vi "settle timer.vi"(2 "in settle band":bool, 7 "Control Parameters":T1={"Setpoint"=50.0, "Control Bandwidth"=4.0, "Integral Time"=30.0, "Int\nON"=TRUE, "Derivative Tme"=0.5, "Der\nON"=TRUE, "Settle Bandwidth"=1.0, "Settle Time"=200.0} {"Settle Time" step=1.0; "Settle Bandwidth" step=0.01; "Derivative Tme" step=0.01; "Integral Time" step=1.0; "Control Bandwidth" step=0.1; "Setpoint" step=0.1}, 9 "reset":bool, 11 "delta t":dbl format="%.2f") -> (8 "time in settle band":dbl format="%.2f", 15 "settled":bool)   [LabVIEW 2019]
doc: "This is a Bug C(T) subVI.\n\nThis VI determines whether the temperature of the system has spent sufficient time in the settle band to deem it settled.\n\nPaul K Dixon\nPhysics 3600\nCSUSB Physics"
uses:
  typedefs/PID control parameters.ctl
panel:
  # "settle timer"
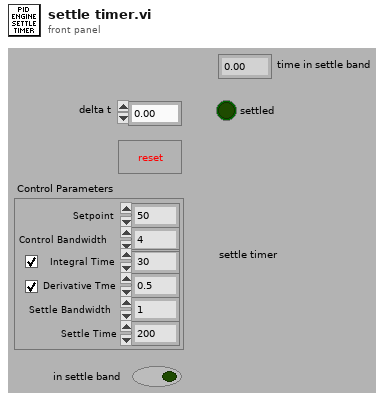
[diagram p1: front panel]
types:
  T1 = typedef "PID control parameters.ctl" = cluster{"Setpoint":dbl, "Control Bandwidth":dbl, "Integral Time":dbl, "Int\nON":bool, "Derivative Tme":dbl, "Der\nON":bool, "Settle Bandwidth":dbl, "Settle Time":dbl}
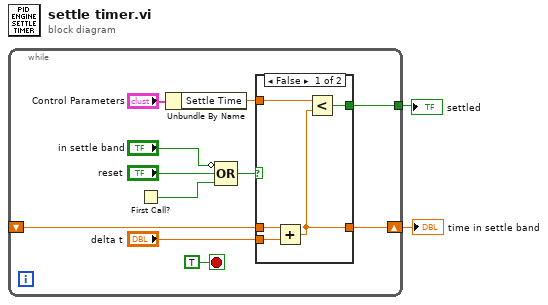
[diagram p0: block diagram]
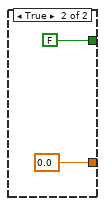
[diagram p2: hidden frame]
diagram:
  n1 = while {
    tunnel: [w5] -> w1
    shift-left: _ -> [w8]
    shift-right: [w9] -> w2
    stop <- TRUE stop-if-true
    n2 = First Call?() -> (First Call?: T/F=w4:bool)
    n3 = Unbundle By Name("Control Parameters") -> ("Settle Time"=w6:dbl)
    n4 = Compound Arithmetic op=OR(invert "in settle band", "reset", w4) -> (w13:bool)
    n5 = case shown="False" w13 {
      tunnel: "delta t" -> [w18 _]
      tunnel: w8 -> [w17 _]
      tunnel: [w15 0.0] -> w9
      tunnel: w6 -> [w16 _]
      tunnel: [w14 FALSE] -> w5
      frame False {
        n6 = Add(x=w17, y=w18) -> (x+y=w15:dbl)
        n7 = Less?(x=w16, y=w15) -> (x < y?=w14:bool)
      }
      frame True {
      }
    }
  }
  "time in settle band" <- w2
  "settled" <- w1
